vi "Parse Owner from Content String.vi"(8 "error in (no error)":errorcluster, 11 "Content string":string) -> (0 "error out":errorcluster, 3 "Owner":T1)   [LabVIEW 2015, in "NI_AWS_S3.lvlib" / "Object.lvlib"]
doc: "Parse out the Owner information from a Content string. Content string is part of the XML string returned by Amazon S3."
uses:
  Object.lvlib
  Owner.ctl
  XML Parsing/NI_XML Parsing.lvlib
  NI_AWS_S3.lvlib
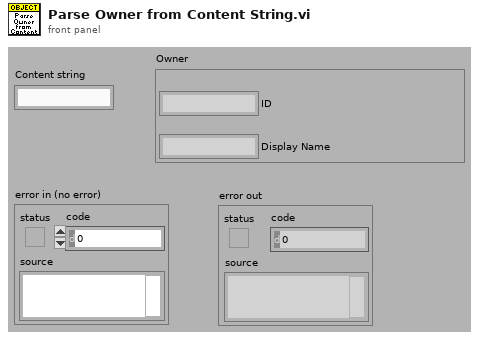
[diagram p1: front panel]
types:
  T1 = typedef "NI_AWS_S3.lvlib/Owner.ctl" = cluster{"ID":string, "Display Name":string}
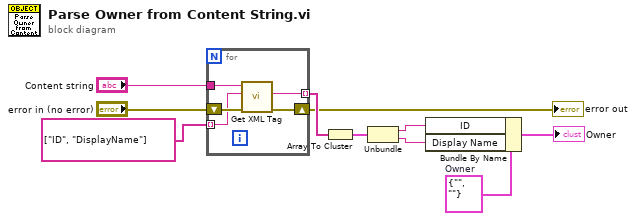
[diagram p0: block diagram]
diagram:
  w10 = T1 {"ID"="", "Display Name"=""}  # Owner
  n1 = for {
    tunnel: string[] ["ID", "DisplayName"] -> [w12] mode=indexing
    shift-right: [w14] -> w4
    shift-left: "error in (no error)" -> [w15]
    tunnel: [w13] -> w8 mode=indexing
    tunnel: "Content string" -> [w11]
    n2 = call "Get XML Tag.vi"("error in (no error)"=w15, "Tag name"=w12, "XML String in"=w11) -> ("error out"=w14:errorcluster, "Tag value"=w13:string)  [unwired: 4 in, 3 out]
  }
  "error out" <- w4
  n3 = Array To Cluster(array=w8) -> (cluster=w7:cluster{"[0]":string, "[1]":string})
  n4 = Unbundle(w7) -> ("[0]"=w5:string, "[1]"=w6:string)
  n5 = Bundle By Name(cluster=w10, "ID"=w5, "Display Name"=w6) -> (→"Owner":T1)
